vi "Help login.vi"() -> ()   [LabVIEW 2018]
panel:
  out "EN help":string="LOGIN\nFor security reasons, only registered users can operate S4ICS. Operations performed by users are recorded for further analysis in the event of an eventual failure.\nUsers get one of the following permissions: Start/Stop, Admin or Control. Only the user with the Admin permission can enter and assign permissions to other users.\nAs long as there is no user registration, S4ICS does not take any action.\n\nOPERATIONAL TIPS\nThe language selector, next to the help button, allows you to hide or show operational tips in available languages. Mouse over the controls and dials to see related tips.\n\nTIMEOUT\nIf the user does not perform any activity for a long time after logging in, S4ICS automatically logs the user out.\n\nBOTTOM WINDOW\nExplanations coming soon." caption="BASIC INFORMATION"
  out "PT help":string="LOGIN\nPor segurança somente usuários cadastrados podem operar o S4ICS. As operações realizadas pelos usuários são registradas para posterior análise no caso de uma falha eventual.\nOs usuários obetm uma das seguintes permissões: Start/Stop, Admin ou Control. Somente o usuário com a permissão Admin pode inserir e atribuir permissões a outros usuários.\nEnquanto não houver o cadastramento de usuários, o S4ICS não executa nenhuma ação.\n\nDICAS DE OPERAÇÃO\nO seletor de idioma, ao lado do botão de ajuda, permite ocultar ou mostrar dicas operacionais nos idiomas disponíveis. Passe o mouse sobre os controles e mostradores para ver as dicas relacionadas. \n\nTIMEOUT\nSe o usuário ficar muito tempo sem executar nenhuma atividade depois de fazer o login, o S4ICS automaticamente faz o logout do usuário.\n\nJANELA INFERIOR\nExplicações em breve.\n" caption="INFORMAÇÕES BÁSICAS"
  in  "ok":bool
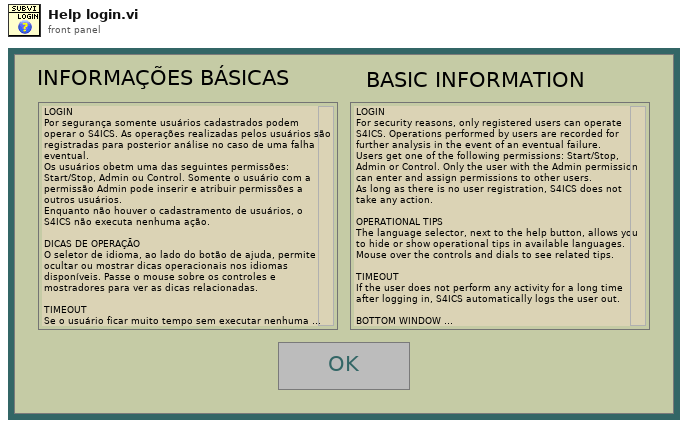
[diagram p1: front panel]
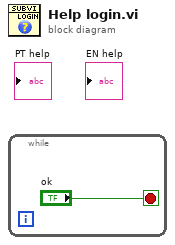
[diagram p0: block diagram]
diagram:
  n1 = while {
    stop <- "ok" stop-if-true
  }
